vi "spring - defer panel updates.vi"(6 "defer panelUpdates (F)":bool, 8 "error in (no error)":errorcluster, 11 "RefNum in":refnum<vi>) -> (0 "error out":errorcluster, 3 "dup RefNum":refnum<vi>)   [LabVIEW 2014]
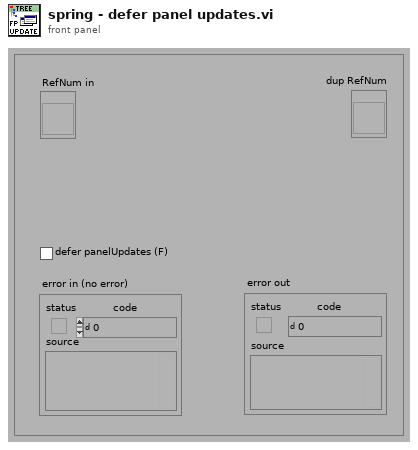
[diagram p1: front panel]
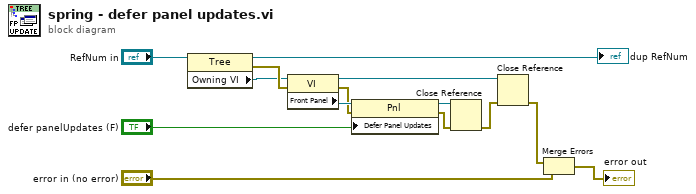
[diagram p0: block diagram]
diagram:
  n1 = property class="Tree"(reference="RefNum in") -> (reference out=→"dup RefNum":refnum<vi>, error out=w13:errorcluster, "Owning VI"=w12:refnum<vi>)  [unwired: 1 in]
  n2 = property class="VI"(reference=w12, error in=w13) -> (reference out=w11:refnum<vi>, error out=w9:errorcluster, "Front Panel"=w10:refnum<vi>)
  n3 = property class="Pnl"(reference=w10, error in=w9, "Defer Panel Updates"="defer panelUpdates (F)") -> (reference out=w8:refnum<vi>, error out=w7:errorcluster)
  n4 = Close Reference(reference=w8, error in (no error)=w7) -> (error out=w6:errorcluster)
  n5 = Close Reference(reference=w11, error in (no error)=w6) -> (error out=w4:errorcluster)
  n6 = Merge Errors(w4, "error in (no error)") -> (→"error out":errorcluster)
